vi "20211217_01.vi"() -> ()   [LabVIEW 2019]
uses:
  <vilib>/regexp/Match Regular Expression.xnode
panel:
  out "after match 2":string
  out "whole match 2":string
  out "before match 2":string
  out "after match":string
  out "before match":string
  out "whole match":string
  out "String":string
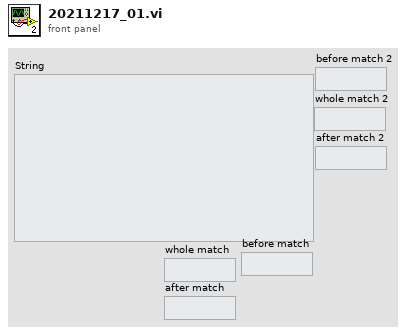
[diagram p1: front panel]
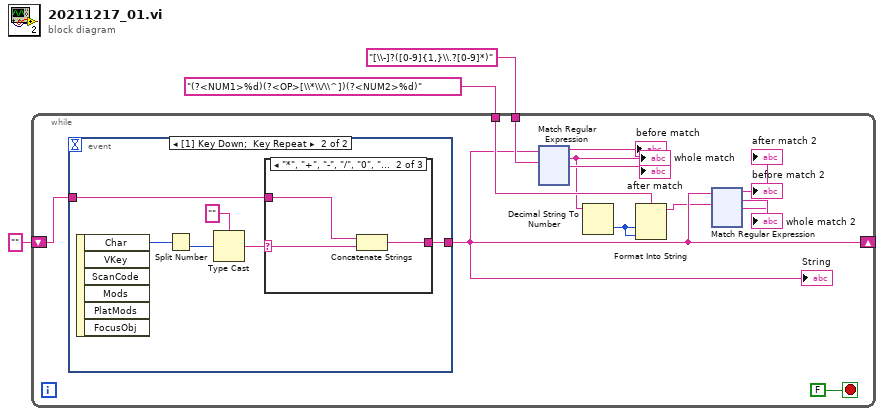
[diagram p0: block diagram]
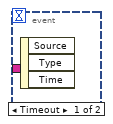
[diagram p2: hidden frame]
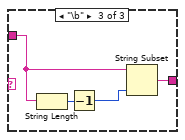
[diagram p4: hidden frame]
diagram:
  n1 = while {
    shift-right: [w8] -> _
    shift-left: "" -> [w15]
    tunnel: "[\\-]?([0-9]{1,}\\.?[0-9]*)" ("regular expression") -> [w12]
    tunnel: "(?<NUM1>%d)(?<OP>[\\*\\/\\^])(?<NUM2>%d)" ("regular expression") -> [w11]
    stop <- FALSE stop-if-true
    n2 = event shown="[1] Key Down;  Key Repeat" {
      selector: _ -> [_ _]
      dyn-events: _ -> [_ _]
      timeout: _ -> [_ _]
      tunnel: [_ w248] -> w8
      tunnel: w15 -> [_ w245]
      event Timeout {
        n3 = event-data() -> ()  [unwired: 1 in, 3 out]
      }
      event Key Down; Key Repeat {
        n4 = event-data() -> ("Char"=w250:i16)  [unwired: 1 in, 5 out]
        n5 = Split Number(x=w250) -> (lo(x)=w249:u8)  [unwired: 1 out]
        n6 = Type Cast(type="", x=w249) -> (*(type *) &x=w246:string)
        n7 = case shown="\"*\", \"+\", \"-\", \"/\", \"0\", \"1\", \"2\", \"3\", \"4\", \"5\", \"6\", \"7\", \"8\", \"9\"" w246 {
          selector: w246 -> [_ w253 _]
          tunnel: [w251 w254 w258] -> w248
          tunnel: w245 -> [w251 w252 w257]
          frame "False", Default {
          }
          frame "*", "+", "-", "/", "0", "1", "2", "3", "4", "5", "6", "7", "8", "9" {
            n8 = Concatenate Strings(w252, w253) -> (w254:string)
          }
          frame "\b" {
            n9 = String Length(string=w257) -> (length=w256:i32)
            n10 = Decrement(x=w256) -> (x-1=w255:i32)
            n11 = String Subset(string=w257, length (rest)=w255) -> (substring=w258:string)  [unwired: 1 in]
          }
        }
      }
    }
    "String" <- w8
    n12 = xnode "Match Regular Expression"("input string"=w8, "regular expression"=w12) -> ("before match"=→"before match":string, "whole match"=w10:string, "after match"=→"after match":string)  [unwired: 4 in, 2 out]
    "whole match" <- w10
    n13 = Decimal String To Number(string=w10) -> (number=w9:i32)  [unwired: 2 in, 1 out]
    n14 = Format Into String(format string=w11, w9, w9) -> (resulting string=w7:string)  [unwired: 2 in, 1 out]
    n15 = xnode "Match Regular Expression"("input string"=w8, "regular expression"=w7) -> ("before match"=→"before match 2":string, "whole match"=→"whole match 2":string, "after match"=→"after match 2":string)  [unwired: 4 in, 2 out]
  }
